vi "Terminate.vi"(8 "error in (no error)":errorcluster, 11 "ATM_UI_Controller in":refnum<class "ATM_UI_Controller.lvclass">) -> (0 "error out":errorcluster, 3 "State out":refnum<class "State Actor.lvclass">)   [LabVIEW 2025, in "ATM_UI_Controller.lvlib" / "ATM_UI_Controller.lvclass"]
uses:
  ATM_UI_Controller.lvclass
  ATM_UI_Controller.lvclass/ATM_UI_Controller.ctl
  C:/Program Files (x86)/National Instruments/LabVIEW 2025/vi.lib/ni/Actors/State Actor/State Actor/State Actor.lvclass
  C:/Program Files (x86)/National Instruments/LabVIEW 2025/vi.lib/ActorFramework/Actor/Actor.lvclass
  C:/Users/halstead_rideriver/Documents/Labview_Practice/ATM_Machine_Actor Framework/ATM_ACTORFW/ATM_UI_Controller/ATM_UI_Controller.lvclass
  Terminate/Terminate.lvclass
  C:/Users/halstead_rideriver/Documents/Labview_Practice/ATM_Machine_Actor Framework/ATM_ACTORFW/ATM_UI_Controller/Terminate/Terminate.lvclass
  <vilib>/ni/Actors/State Actor/State Actor/State Actor.lvclass
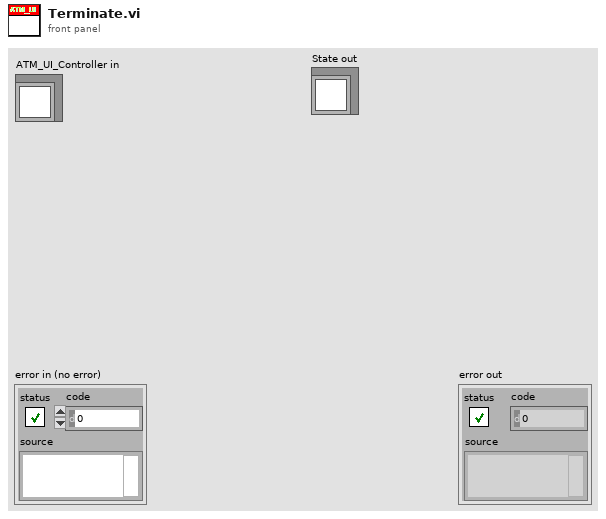
[diagram p1: front panel]
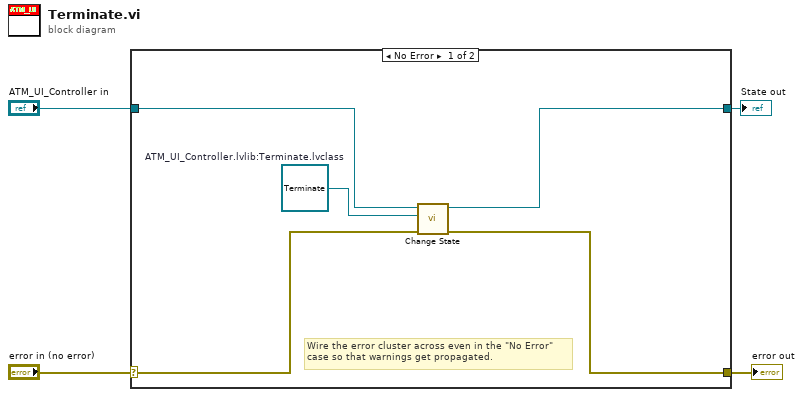
[diagram p0: block diagram]
diagram:
  n1 = case shown="No Error" "error in (no error)" {
    selector: "error in (no error)" -> [w8 w11]
    tunnel: [w7 w11] -> w3
    tunnel: [w6 w10] -> w1
    tunnel: "ATM_UI_Controller in" -> [w9 w10]
    frame No Error {
      w5 = refnum<class "Terminate.lvclass"> refnum  # ATM_UI_Controller.lvlib:Terminate.lvclass
      # "Wire the error cluster across even in the \"No Error\"\ncase so that warnings get propagated."
      n2 = call <vilib>:"Change State.vi"("error in (no error)"=w8, "New State in"=w5, "State in"=w9) -> ("error out"=w7:errorcluster, "State out"=w6:refnum<class "State Actor.lvclass">)  [unwired: 7 in]
    }
    frame Error {
    }
  }
  "error out" <- w3
  "State out" <- w1
